vi "Drive Train Update Metrics.vi"(10 "Input":T1) -> (2 "Output":T1)   [LabVIEW 2014]
uses:
  Drive Train Metrics.ctl
  CmdFlag.ctl
panel:
  out "Right Distance":dbl(graph)
  out "Left Distance":dbl(graph)
  out "Right Rate":dbl(graph)
  out "Left Rate":dbl(graph)
  out "Acceleration":dbl(graph)
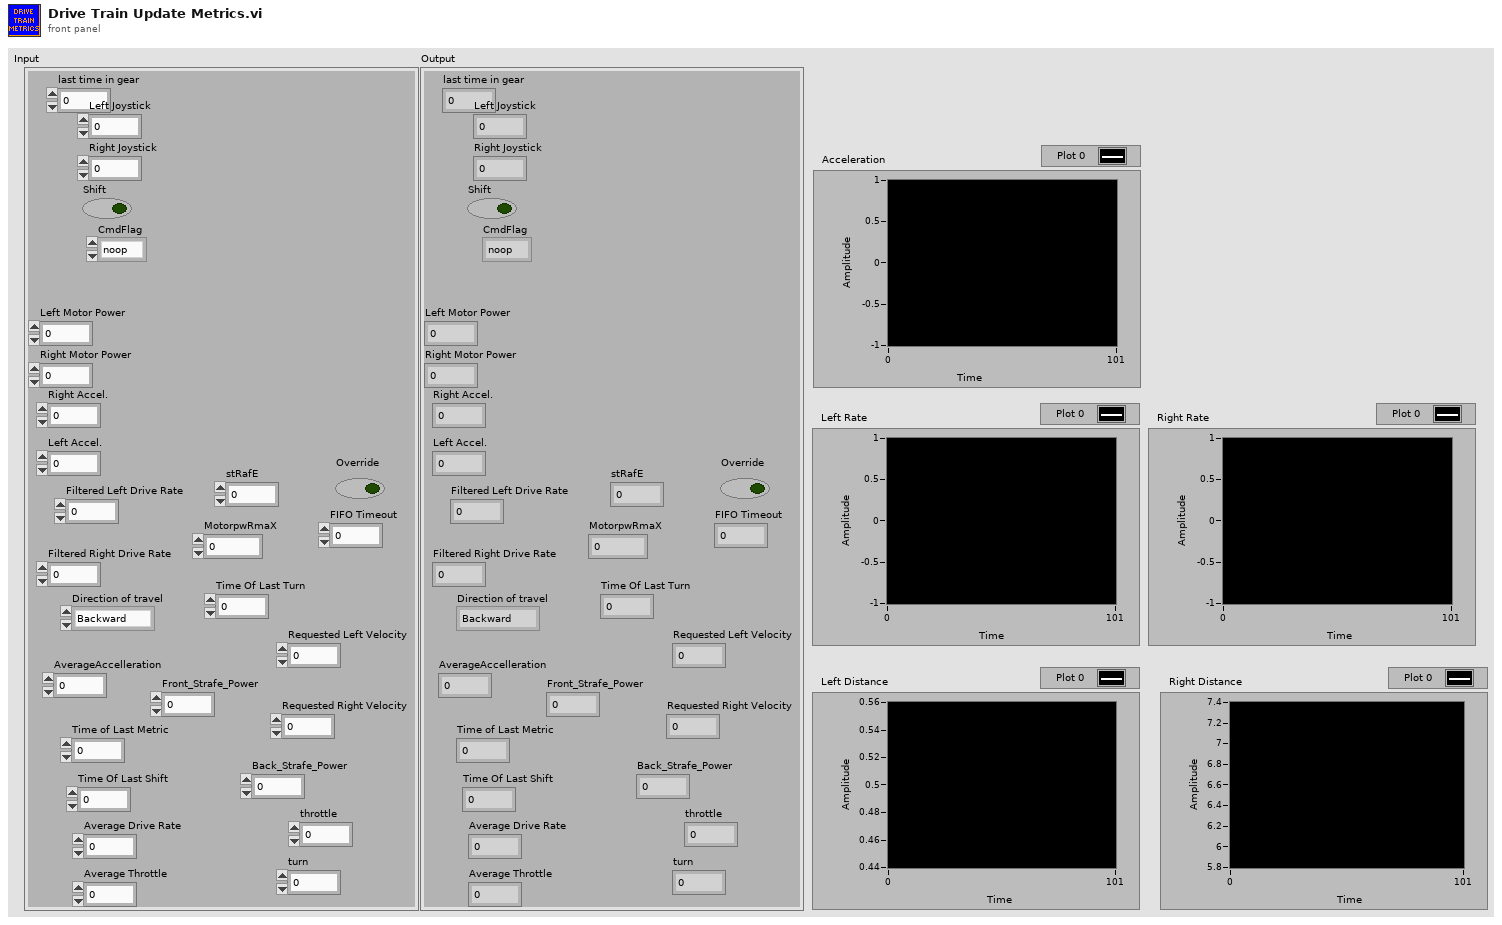
[diagram p1: front panel]
types:
  T1 = typedef "Drive Train Metrics.ctl" = cluster{"last time in gear":u32, "Shift":bool, "Right Joystick":dbl, "Left Joystick":dbl, "CmdFlag":T2, "Right Motor Power":dbl, "Left Motor Power":dbl, "Right Accel.":dbl, "Left Accel.":dbl, "Filtered Left Drive Rate":dbl, "Filtered Right Drive Rate":dbl, "Direction of travel":enum16{"Backward", "Forward", "Spin"}, "AverageAccelleration":dbl, "Time of Last Metric":u32, "Time Of Last Shift":dbl, "Average Drive Rate":dbl, "Average Throttle":dbl, "FIFO Timeout":i32, "Requested Left Velocity":dbl, "Requested Right Velocity":dbl, "throttle":dbl, "turn":dbl, "MotorpwRmaX":i32, "stRafE":i32, "Override":bool, "Time Of Last Turn":dbl, "Front_Strafe_Power":dbl, "Back_Strafe_Power":dbl}
  T2 = typedef "CmdFlag.ctl" = enum16{"noop", "suspend", "resume"}
  T3 = typedef "WPI_EncoderDevRef.ctl" = cluster{"DevStatus":errorcluster, "EncoderIndex":T4, "CounterIndex":T5, "DistancePerCount":dbl, "Decoding Type":T6}
  T4 = typedef "FPGA_EncoderIdx.ctl" = enum8{"Enc 0", "Enc 1", "Enc 2", "Enc 3", "Enc 4", "Enc 5", "Enc 6", "Enc 7", "Invalid"}
  T5 = typedef "FPGA_CounterCtrSystemIndex.ctl" = enum8{"Ctr 0", "Ctr 1", "Ctr 2", "Ctr 3", "Ctr 4", "Ctr 5", "Ctr 6", "Ctr 7", "Invalid"}
  T6 = typedef "WPI_EncoderType.ctl" = enum16{"1x", "2x", "4x"}
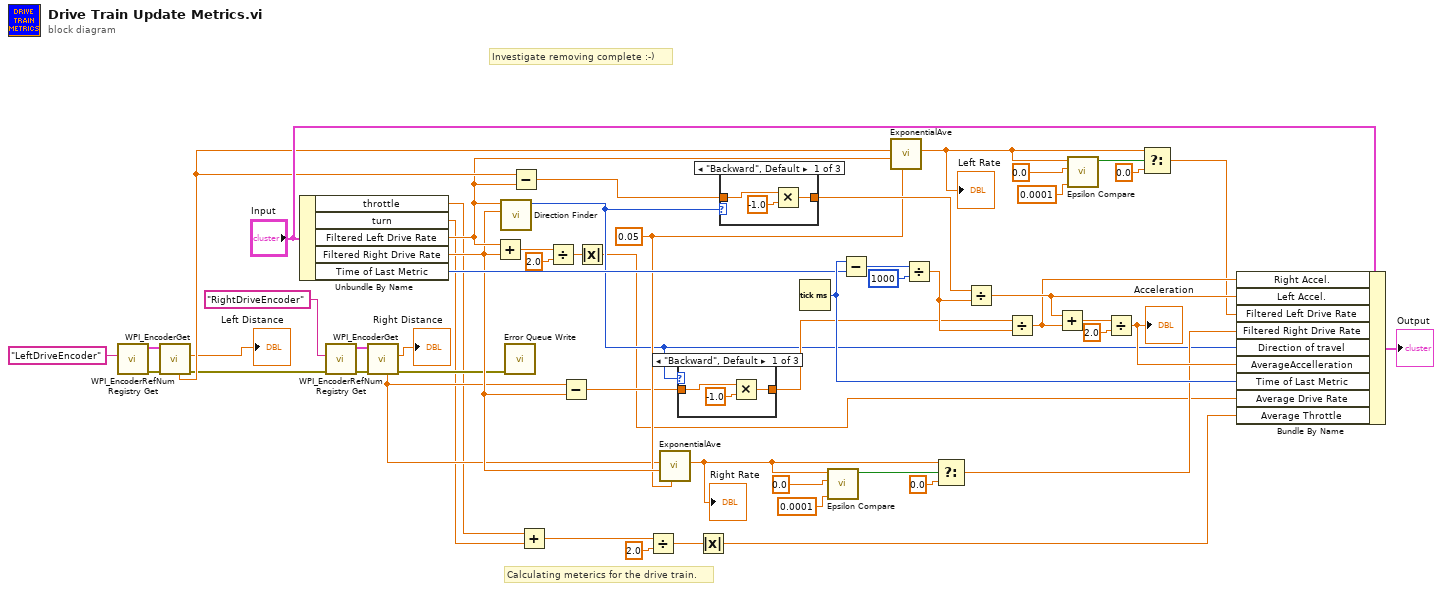
[diagram p0: block diagram]
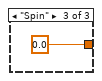
[diagram p3: hidden frame]
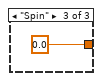
[diagram p5: hidden frame]
diagram:
  w26 = 0.05 ("Coff")
  # "Investigate removing complete :-)"
  # "Calculating meterics for the drive train."
  n1 = call <vilib>:"WPI_EncoderRefNum Registry Get.vi"("refnum name"="LeftDriveEncoder") -> ("error out"=w53:errorcluster, "EncoderDevRef"=w52:T3)  [unwired: 9 in]
  n2 = call <vilib>:"WPI_EncoderGet.vi"("error in (no error)"=w53, "EncoderDevRef"=w52) -> ("error out"=w7:errorcluster, "Distance"=→"Left Distance":dbl, "Rate"=w36:dbl)  [unwired: 4 in, 3 out]
  n3 = Unbundle By Name("Input") -> ("throttle"=w6:dbl, "turn"=w5:dbl, "Filtered Left Drive Rate"=w31:dbl, "Filtered Right Drive Rate"=w30:dbl, "Time of Last Metric"=w41:u32)
  n4 = call <vilib>:"WPI_EncoderRefNum Registry Get.vi"("error in (no error)"=w7, "refnum name"="RightDriveEncoder") -> ("error out"=w50:errorcluster, "EncoderDevRef"=w49:T3)  [unwired: 8 in]
  n5 = call <vilib>:"WPI_EncoderGet.vi"("error in (no error)"=w50, "EncoderDevRef"=w49) -> ("error out"=w8:errorcluster, "Distance"=→"Right Distance":dbl, "Rate"=w9:dbl)  [unwired: 4 in, 3 out]
  n6 = Add(x=w31, y=w30) -> (x+y=w32:dbl)
  n7 = call "Direction Finder.vi"("Filtered Right Drive Rate"=w30, "Filtered Left Drive Rate"=w31) -> ("Direction of travel"=w2:enum16{"Backward", "Forward", "Spin"})  [unwired: 9 in]
  n8 = call "Error Queue Write.vi"("error in (no error)"=w8) -> ()  [unwired: 11 in]
  n9 = Subtract(x=w36, y=w31) -> (x-y=w46:dbl)
  n10 = Add(x=w6, y=w5) -> (x+y=w25:dbl)
  n11 = Divide(x=w32, y=2.0) -> (x/y=w29:dbl)
  n12 = Subtract(x=w9, y=w30) -> (x-y=w3:dbl)
  n13 = Absolute Value(x=w29) -> (abs(x)=w1:dbl)
  n14 = Divide(x=w25, y=2.0) -> (x/y=w23:dbl)
  n15 = call "ExponentialAve.vi"("Coff"=w26, "PreviousValue"=w30, "InputValue"=w9) -> ("Smoothed Value"=w11:dbl)  [unwired: 8 in]
  "Right Rate" <- w11
  n16 = case shown="\"Backward\", Default" w2 {
    tunnel: [w55 w58 0.0] -> w4
    tunnel: w3 -> [w56 w58 _]
    frame "Backward", Default {
      n17 = Multiply(x=w56, y=-1.0) -> (x*y=w55:dbl)
    }
    frame "Forward" {
    }
    frame "Spin" {
    }
  }
  n18 = Absolute Value(x=w23) -> (abs(x)=w22:dbl)
  n19 = case shown="\"Backward\", Default" w2 {
    tunnel: [w60 w63 0.0] -> w40
    tunnel: w46 -> [w61 w63 _]
    frame "Backward", Default {
      n20 = Multiply(x=w61, y=-1.0) -> (x*y=w60:dbl)
    }
    frame "Forward" {
    }
    frame "Spin" {
    }
  }
  n21 = Tick Count (ms)() -> (millisecond timer value=w42:u32)
  n22 = call "Epsilon Compare.vi"("Epsilon"=0.0001, "Value2"=0.0, "Value1"=w11) -> ("Boolean"=w13:bool)  [unwired: 8 in]
  n23 = Subtract(x=w42, y=w41) -> (x-y=w39:u32)
  n24 = call "ExponentialAve.vi"("Coff"=w26, "PreviousValue"=w31, "InputValue"=w36) -> ("Smoothed Value"=w18:dbl)  [unwired: 8 in]
  "Left Rate" <- w18
  n25 = Divide(x=w39, y=u32 1000) -> (x/y=w28:dbl)
  n26 = Select(t=w11, s=w13, f=0.0) -> (s? t:f=w10:dbl)
  n27 = Divide(x=w40, y=w28) -> (x/y=w38:dbl)
  n28 = Divide(x=w4, y=w28) -> (x/y=w37:dbl)
  n29 = Add(x=w38, y=w37) -> (x+y=w45:dbl)
  n30 = call "Epsilon Compare.vi"("Epsilon"=0.0001, "Value2"=0.0, "Value1"=w18) -> ("Boolean"=w19:bool)  [unwired: 8 in]
  n31 = Divide(x=w45, y=2.0) -> (x/y=w43:dbl)
  "Acceleration" <- w43
  n32 = Select(t=w18, s=w19, f=0.0) -> (s? t:f=w16:dbl)
  n33 = Bundle By Name(cluster="Input", "Right Accel."=w37, "Left Accel."=w38, "Filtered Left Drive Rate"=w16, "Filtered Right Drive Rate"=w10, "Direction of travel"=w2, "AverageAccelleration"=w43, "Time of Last Metric"=w42, "Average Drive Rate"=w1, "Average Throttle"=w22) -> (→"Output":T1)
